vi "Check List.vi"(8 "Channel Data in":T1, 9 "Parent Tag":string, 10 "Sh Var URL":string, 11 "List in":T3[](array[typedef])) -> (0 "Channel Data out":T1, 2 "Found?":bool, 3 "List out":T3[](array[typedef]))   [LabVIEW 2015, in "Shared Variable Custom Device.lvlib"]
uses:
  Shared Variable Custom Device.lvlib
  Tree Data.ctl
  <vilib>/Utility/VariantDataType/Type.ctl
  Existing Channel Data.ctl
  <vilib>/Utility/VariantDataType/VariantType.lvlib
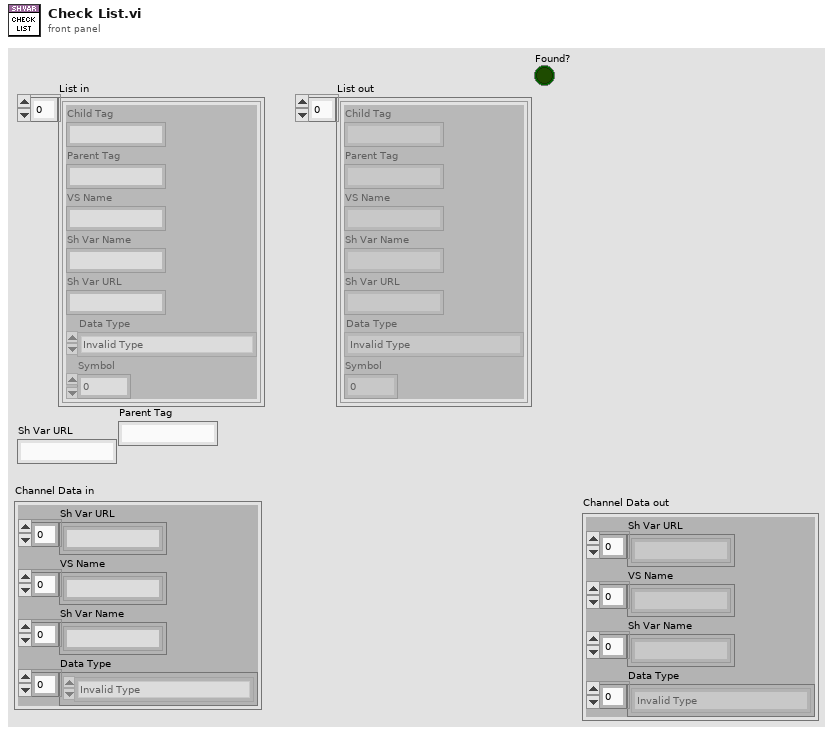
[diagram p1: front panel]
types:
  T1 = typedef "Shared Variable Custom Device.lvlib/Existing Channel Data.ctl" = cluster{"Sh Var URL":string[], "VS Name":string[], "Sh Var Name":string[], "Data Type":T2[]}
  T2 = typedef "VariantType.lvlib/Type.ctl" = enum8{"Invalid Type", "Void", "I8", "I16", "I32", "I64", "U8", "U16", "U32", "U64", "Single Float", "Double Float", "Extended Float", "Single Complex", "Double Complex", "Extended Complex", "Enum U8", "Enum U16", "Enum U32", "Enum U64", "Single Float With Unit", "Double Float With Unit", "Extended Float With Unit", "Single Complex with Unit", "Double Complex with Unit", "Extended Complex with Unit", "Boolean", "String", "Path", "Picture", "Tag", "Array", "Cluster", "Variant", "LV Variant", "Waveform", "Timestamp", "Digital Waveform", "Digital Data", "ExpressData", "Refnum", "External Data", "VI", "Poly VI", "LabVIEW Class Instance", "Fixed Point"}
  T3 = typedef "Shared Variable Custom Device.lvlib/Tree Data.ctl" = cluster{"Child Tag":string, "Parent Tag":string, "VS Name":string, "Sh Var Name":string, "Sh Var URL":string, "Data Type":T2, "Symbol":i32}
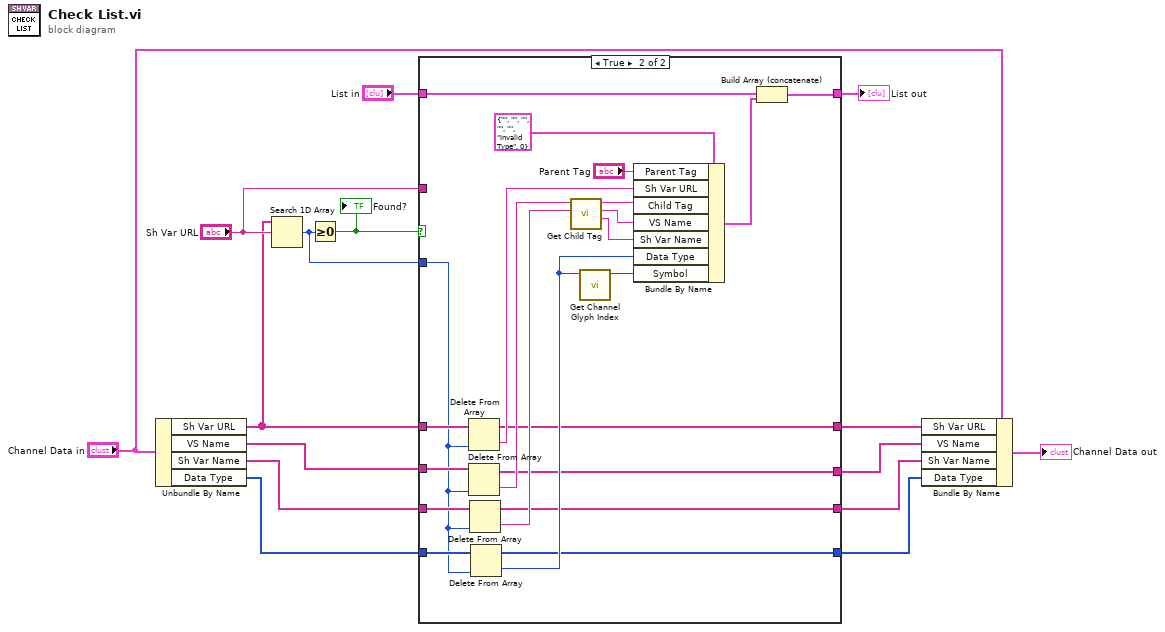
[diagram p0: block diagram]
diagram:
  n1 = Unbundle By Name("Channel Data in") -> ("Sh Var URL"=w2:string[], "VS Name"=w10:string[], "Sh Var Name"=w9:string[], "Data Type"=w8:T2[])
  n2 = Search 1D Array(1D array=w2, element="Sh Var URL") -> (index of element=w14:i32)  [unwired: 1 in]
  n3 = Greater Or Equal To 0?(x=w14) -> (x >= 0?=w11:bool)
  "Found?" <- w11
  n4 = case shown="True" w11 {
    tunnel: "List in" -> [w20 w42]
    tunnel: [w20 w41] -> w13
    tunnel: w8 -> [w17 w30]
    tunnel: w10 -> [w19 w37]
    tunnel: w14 -> [_ w23]
    tunnel: w9 -> [w18 w32]
    tunnel: [w17 w28] -> w3
    tunnel: "Sh Var URL" -> [_ _]
    tunnel: [w18 w27] -> w4
    tunnel: [w19 w26] -> w5
    tunnel: w2 -> [w16 w24]
    tunnel: [w16 w21] -> w1
    frame False {
    }
    frame True {
      n5 = Delete From Array(array=w24, index=w23) -> (deleted portion=w22:string, array with subset deleted=w21:string[])  [unwired: 1 in]
      n6 = Delete From Array(array=w37, index=w23) -> (deleted portion=w36:string, array with subset deleted=w26:string[])  [unwired: 1 in]
      n7 = Delete From Array(array=w32, index=w23) -> (deleted portion=w31:string, array with subset deleted=w27:string[])  [unwired: 1 in]
      n8 = Delete From Array(array=w30, index=w23) -> (deleted portion=w29:T2, array with subset deleted=w28:T2[])  [unwired: 1 in]
      n9 = call "Get Child Tag.vi"("Sh Var Name in"=w31, "VS Name in"=w36) -> ("Sh Var Name out"=w33:string, "VS Name out"=w34:string, "Child Tag"=w35:string)  [unwired: 7 in]
      n10 = call "Get Channel Glyph Index.vi"("Channel Type"=w29) -> ("Glyph Index"=w39:i32)  [unwired: 10 in]
      n11 = Bundle By Name(cluster=T3 {"Child Tag"="", "Parent Tag"="", "VS Name"="", "Sh Var Name"="", "Sh Var URL"="", "Data Type"=enum."Invalid Type", "Symbol"=0} ("Tree Data"), "Parent Tag"="Parent Tag", "Sh Var URL"=w22, "Child Tag"=w35, "VS Name"=w34, "Sh Var Name"=w33, "Data Type"=w29, "Symbol"=w39) -> (w38:T3)
      n12 = Build Array (concatenate)(w42, w38) -> (w41:T3[])
    }
  }
  "List out" <- w13
  n13 = Bundle By Name(cluster="Channel Data in", "Sh Var URL"=w1, "VS Name"=w5, "Sh Var Name"=w4, "Data Type"=w3) -> (→"Channel Data out":T1)
